vi "sensor config get label v2.vi"(7 "buff_size":i32, 9 "BYTE_ARRAY":string, 10 "label_string":u32(ring) items=["CONFIG_V2_STRING_LABEL_0", "CONFIG_V2_STRING_LABEL_1", "CONFIG_V2_STRING_LABEL_2", "CONFIG_V2_STRING_LOCATION", "CONFIG_V2_STRING_TIMEZONE", "CONFIG_V2_STRING_BUTTON_EVENT_0", "CONFIG_V2_STRING_BUTTON_EVENT_1", "CONFIG_V2_STRING_BUTTON_EVENT_2", "CONFIG_V2_STRING_BUTTON_EVENT_3", "CONFIG_V2_STRING_TIMEZONE_OFFSET", "CONFIG_V2_STRING_LAST_VALUE"], 11 "device_handle":u32) -> (1 "BYTE_ARRAY out":string, 2 "function return":i32, 3 "device_handle out":u32)   [LabVIEW 2019, in "apdm.lvlib"]
doc: "APDM_EXPORT int apdm_sensor_config_get_label_v2(apdm_device_handle_t device_handle, const config_v2_string_t label_string, char *BYTE_ARRAY, const int buff_size);"
uses:
  apdm.lvlib
  Lee Lab/CP FES Walking 2018/Code/Working/LabVIEW/apdm.dll
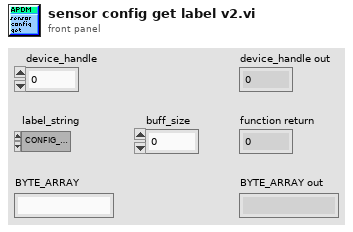
[diagram p1: front panel]
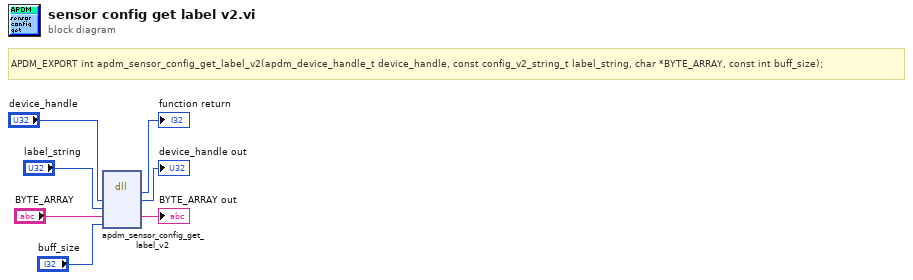
[diagram p0: block diagram]
diagram:
  # "APDM_EXPORT int apdm_sensor_config_get_label_v2(apdm_device_handle_t device_handle, const config_v2_string_t label_string, char *BYTE_ARRAY, const int buff_size);"
  n1 = dll-call lib="C:/Users/jfalesi/Dropbox/Lee Lab/CP FES Walking 2018/Code/Working/LabVIEW/apdm.*" fn="apdm_sensor_config_get_label_v2"("device_handle"="device_handle", "label_string"="label_string", "BYTE_ARRAY"="BYTE_ARRAY", "buff_size"="buff_size") -> (→"function return":i32, "device_handle"=→"device_handle out":u32, "BYTE_ARRAY"=→"BYTE_ARRAY out":string)  [unwired: 5 in, 2 out]
